vi "Large integer U8 array - multiply by constant.vi"(3 "Constant U8":u8, 5 "Large number - U8":T1) -> (1 "Multiplied array":T1)   [LabVIEW 2012]
doc: "Multiplies a large numbers (U8 array format) by a constant U8"
uses:
  User Access Type defs/Large number - U8 array.ctl
panel:
  # "index 0 = LSD"
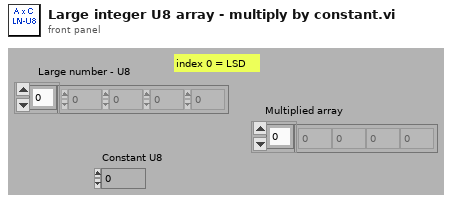
[diagram p1: front panel]
types:
  T1 = typedef "Large number - U8 array.ctl" = u8[]
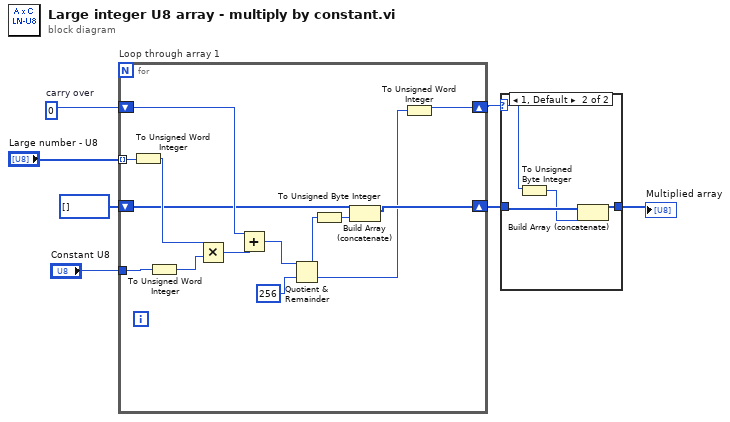
[diagram p0: block diagram]
diagram:
  w4 = u16 0  # carry over
  n1 = for "Loop through array 1" {
    shift-right: [w11] -> w2
    shift-left: T1 [] ("Added array") -> [w13]
    tunnel: "Large number - U8" -> [w21] mode=indexing
    tunnel: "Constant U8" -> [w18]
    shift-right: [w8] -> w3
    shift-left: w4 -> [w15]
    n2 = To Unsigned Word Integer(number=w21) -> (unsigned 16bit integer=w20:u16)
    n3 = To Unsigned Word Integer(number=w18) -> (unsigned 16bit integer=w19:u16)
    n4 = Multiply(x=w20, y=w19) -> (x*y=w16:u16)
    n5 = Add(x=w15, y=w16) -> (x+y=w14:u16)
    n6 = Quotient & Remainder(x=w14, y=u16 256) -> (x-y*floor(x/y)=w12:u16, floor(x/y)=w9:u16)
    n7 = To Unsigned Byte Integer(number=w12) -> (unsigned 8bit integer=w10:u8)
    n8 = Build Array (concatenate)(w13, w10) -> (w11:T1)
    n9 = To Unsigned Word Integer(number=w9) -> (unsigned 16bit integer=w8:u16)
  }
  n10 = case shown="1, Default" w3 {
    selector: w3 -> [_ w25]
    tunnel: [w22 w23] -> w1
    tunnel: w2 -> [w22 w26]
    frame 0 {
    }
    frame 1, Default {
      n11 = To Unsigned Byte Integer(number=w25) -> (unsigned 8bit integer=w24:u8)
      n12 = Build Array (concatenate)(w26, w24) -> (w23:T1)
    }
  }
  "Multiplied array" <- w1
